vi "Pracownia5.vi"() -> ()   [LabVIEW 2019]
panel:
  out "Liczba binarnie":bool[](array[boolean])
  in  "Zero":bool
  in  "Liczba":u8
  in  "stop":bool
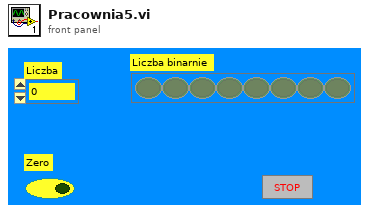
[diagram p1: front panel]
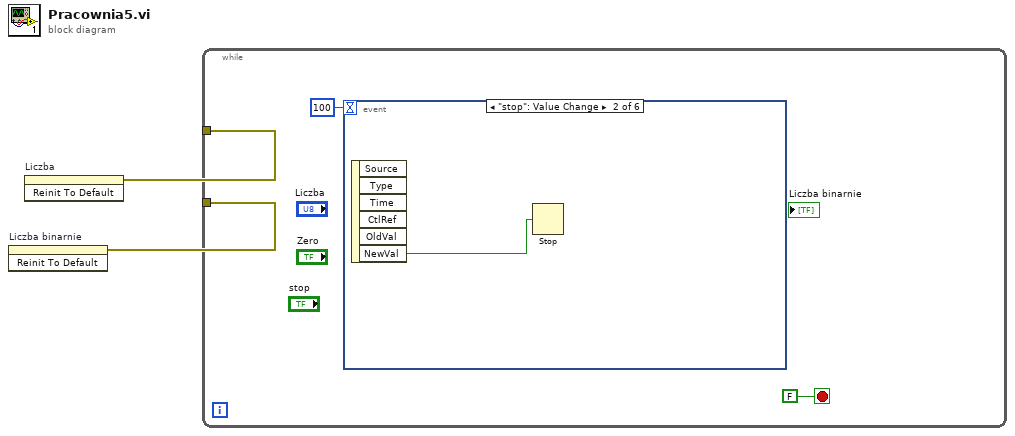
[diagram p0: block diagram]
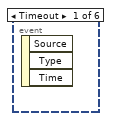
[diagram p2: hidden frame]
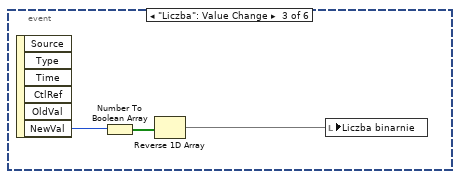
[diagram p3: hidden frame]
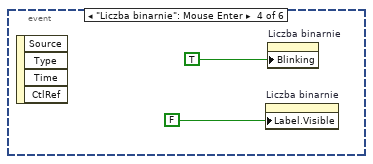
[diagram p4: hidden frame]
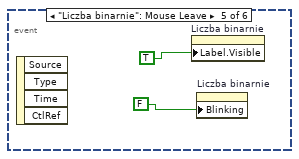
[diagram p5: hidden frame]
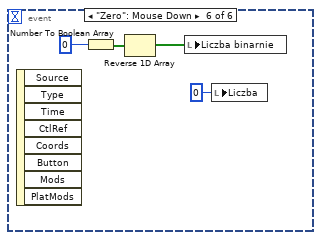
[diagram p6: hidden frame]
diagram:
  n1 = invoke on="Liczba binarnie" class="Arr (strict)" method="Reinit To Default"() -> (error out=w2:errorcluster)  [unwired: 3 in, 2 out]
  n2 = invoke on="Liczba" class="DigNum (strict)" method="Reinit To Default"() -> (error out=w1:errorcluster)  [unwired: 3 in, 2 out]
  n3 = while {
    tunnel: w2 -> [_]
    tunnel: w1 -> [_]
    stop <- FALSE stop-if-true
    n4 = event shown="[1] \"stop\": Value Change" {
      selector: _ -> [_ _ _ _ _ _]
      dyn-events: _ -> [_ _ _ _ _ _]
      timeout: 100 -> [_ _ _ _ _ _]
      event Timeout {
        n5 = event-data() -> ()  [unwired: 1 in, 3 out]
      }
      event "stop": Value Change {
        n6 = event-data() -> ("NewVal"=w5:bool)  [unwired: 1 in, 5 out]
        n7 = Stop(stop? (T)=w5) -> ()
      }
      event "Liczba": Value Change {
        n8 = event-data() -> ("NewVal"=w8:u8)  [unwired: 1 in, 5 out]
        n9 = Number To Boolean Array(number=w8) -> (Boolean array=w7:bool[])
        n10 = Reverse 1D Array(array=w7) -> (reversed array=w6:bool[])
        n11 = local write "Liczba binarnie"(w6) -> ()
      }
      event "Liczba binarnie": Mouse Enter {
        n12 = event-data() -> ()  [unwired: 1 in, 4 out]
        n13 = property on="Liczba binarnie" class="Arr (strict)"("Label.Visible"=FALSE) -> ()  [unwired: 2 in, 2 out]
        n14 = property on="Liczba binarnie" class="Arr (strict)"("Blinking"=TRUE) -> ()  [unwired: 2 in, 2 out]
      }
      event "Liczba binarnie": Mouse Leave {
        n15 = event-data() -> ()  [unwired: 1 in, 4 out]
        n16 = property on="Liczba binarnie" class="Arr (strict)"("Label.Visible"=TRUE) -> ()  [unwired: 2 in, 2 out]
        n17 = property on="Liczba binarnie" class="Arr (strict)"("Blinking"=FALSE) -> ()  [unwired: 2 in, 2 out]
      }
      event "Zero": Mouse Down {
        n18 = event-data() -> ()  [unwired: 1 in, 8 out]
        n19 = Number To Boolean Array(number=u8 0) -> (Boolean array=w14:bool[])
        n20 = Reverse 1D Array(array=w14) -> (reversed array=w13:bool[])
        n21 = local write "Liczba binarnie"(w13) -> ()
        n22 = local write "Liczba"(u8 0 ("Liczba")) -> ()
      }
    }
  }
